vi "Update Measurement from Metadata.vi"(7 "client service_class":string, 8 "error in":errorcluster, 9 "default value":variant, 10 "metadata":T1, 11 "file refnums":refnum<vi>[](array[refnum])) -> (0 "error out":errorcluster)   [LabVIEW 2021, in "NI Measurement V2 Client Generator Runtime.lvlib"]
uses:
  NI Measurement V2 Client Generator Runtime.lvlib
  <vilib>/gRPC/Generated APIs/ni/measurementlink/measurement/v2/Measurement Service Client V2/RPC Messages/ni_measurementlink_measurement_v2_GetMetadataResponse.ctl
  <vilib>/gRPC/Generated APIs/ni/measurementlink/measurement/v2/Measurement Service Client V2/RPC Messages/ni_measurementlink_measurement_v2_MeasurementDetails.ctl
  <vilib>/gRPC/Generated APIs/ni/measurementlink/measurement/v2/Measurement Service Client V2/RPC Messages/ni_measurementlink_measurement_v2_MeasurementSignature.ctl
  <vilib>/gRPC/Generated APIs/ni/measurementlink/measurement/v2/Measurement Service Client V2/RPC Messages/ni_measurementlink_measurement_v2_ConfigurationParameter.ctl
  <vilib>/gRPC/Generated APIs/ni/measurementlink/measurement/v2/Measurement Service Client V2/RPC Messages/google_protobuf_Field_Kind.ctl
  <vilib>/gRPC/Generated APIs/ni/measurementlink/measurement/v2/Measurement Service Client V2/RPC Messages/ni_measurementlink_measurement_v2_ConfigurationParameter_AnnotationsEntry.ctl
  <vilib>/gRPC/Generated APIs/ni/measurementlink/measurement/v2/Measurement Service Client V2/RPC Messages/google_protobuf_Any.ctl
  <vilib>/gRPC/Generated APIs/ni/measurementlink/measurement/v2/Measurement Service Client V2/RPC Messages/ni_measurementlink_measurement_v2_Output.ctl
  <vilib>/gRPC/Generated APIs/ni/measurementlink/measurement/v2/Measurement Service Client V2/RPC Messages/ni_measurementlink_measurement_v2_Output_AnnotationsEntry.ctl
  <vilib>/gRPC/Generated APIs/ni/measurementlink/measurement/v2/Measurement Service Client V2/RPC Messages/ni_measurementlink_measurement_v2_UserInterfaceDetails.ctl
  <vilib>/Utility/traverseref.llb/TRef TravTarget.ctl
  Client Generator Error Strings Global.vi
  <vilib>/Utility/traverseref.llb/VI Scripting - Traverse.lvlib
  <vilib>/gRPC/Generated APIs/ni/measurementlink/measurement/v2/Measurement Service Client V2/Measurement Service Client V2.lvlib
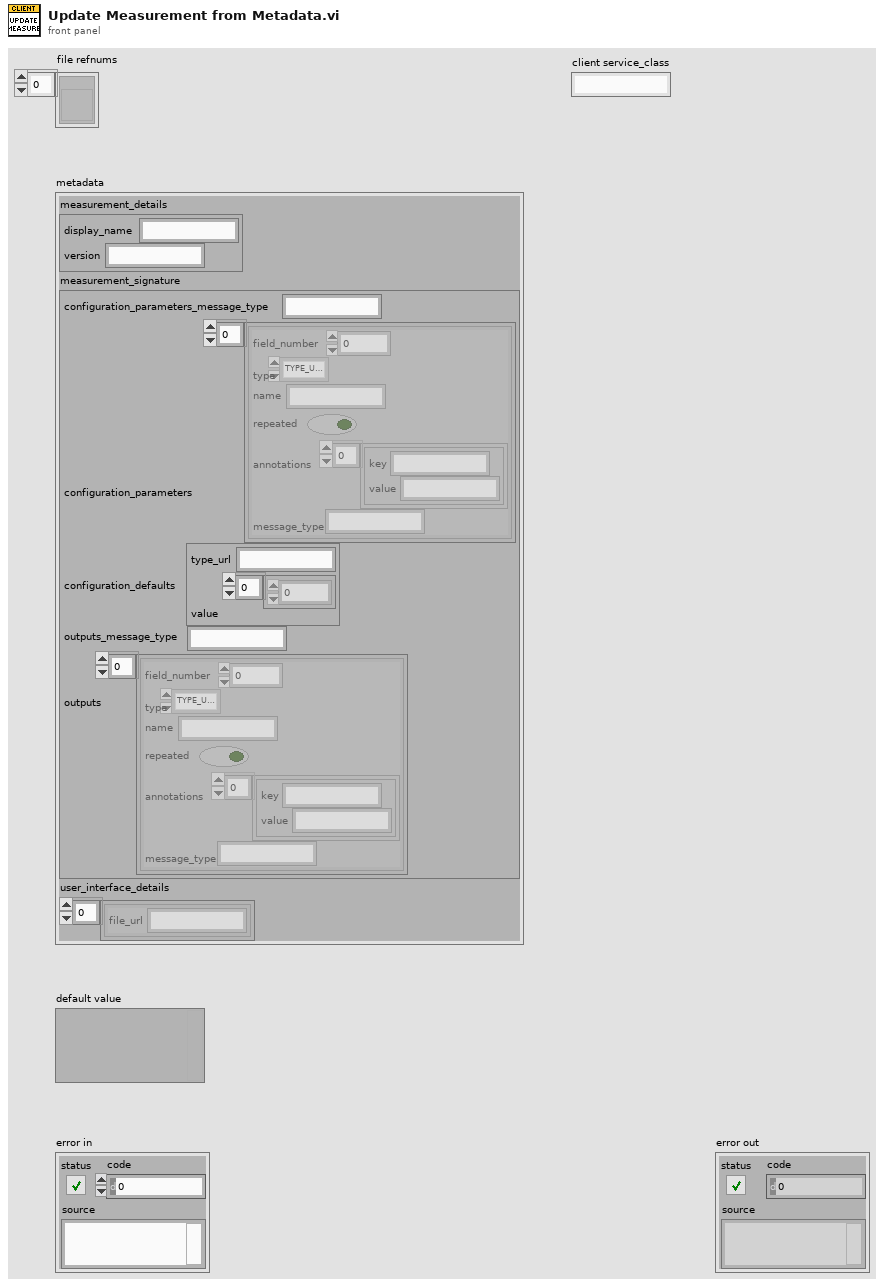
[diagram p1: front panel]
types:
  T1 = typedef "Measurement Service Client V2.lvlib/ni_measurementlink_measurement_v2_GetMetadataResponse.ctl" = cluster{"measurement_details":T2, "measurement_signature":T3, "user_interface_details":T10[]}
  T2 = typedef "Measurement Service Client V2.lvlib/ni_measurementlink_measurement_v2_MeasurementDetails.ctl" = cluster{"display_name":string, "version":string}
  T3 = typedef "Measurement Service Client V2.lvlib/ni_measurementlink_measurement_v2_MeasurementSignature.ctl" = cluster{"configuration_parameters_message_type":string, "configuration_parameters":T4[], "configuration_defaults":T7, "outputs_message_type":string, "outputs":T8[]}
  T4 = typedef "Measurement Service Client V2.lvlib/ni_measurementlink_measurement_v2_ConfigurationParameter.ctl" = cluster{"field_number":i32, "type":T5, "name":string, "repeated":bool, "annotations":T6[], "message_type":string}
  T5 = typedef "Measurement Service Client V2.lvlib/google_protobuf_Field_Kind.ctl" = enum32{"TYPE_UNKNOWN", "TYPE_DOUBLE", "TYPE_FLOAT", "TYPE_INT64", "TYPE_UINT64", "TYPE_INT32", "TYPE_FIXED64", "TYPE_FIXED32", "TYPE_BOOL", "TYPE_STRING", "TYPE_GROUP", "TYPE_MESSAGE", "TYPE_BYTES", "TYPE_UINT32", "TYPE_ENUM", "TYPE_SFIXED32", "TYPE_SFIXED64", "TYPE_SINT32", "TYPE_SINT64"}
  T6 = typedef "Measurement Service Client V2.lvlib/ni_measurementlink_measurement_v2_ConfigurationParameter_AnnotationsEntry.ctl" = cluster{"key":string, "value":string}
  T7 = typedef "Measurement Service Client V2.lvlib/google_protobuf_Any.ctl" = cluster{"type_url":string, "value":u8[]}
  T8 = typedef "Measurement Service Client V2.lvlib/ni_measurementlink_measurement_v2_Output.ctl" = cluster{"field_number":i32, "type":T5, "name":string, "repeated":bool, "annotations":T9[], "message_type":string}
  T9 = typedef "Measurement Service Client V2.lvlib/ni_measurementlink_measurement_v2_Output_AnnotationsEntry.ctl" = cluster{"key":string, "value":string}
  T10 = typedef "Measurement Service Client V2.lvlib/ni_measurementlink_measurement_v2_UserInterfaceDetails.ctl" = cluster{"file_url":string}
  T11 = typedef "TRef TravTarget.ctl" = enum16{"FP", "BD", "Other"}
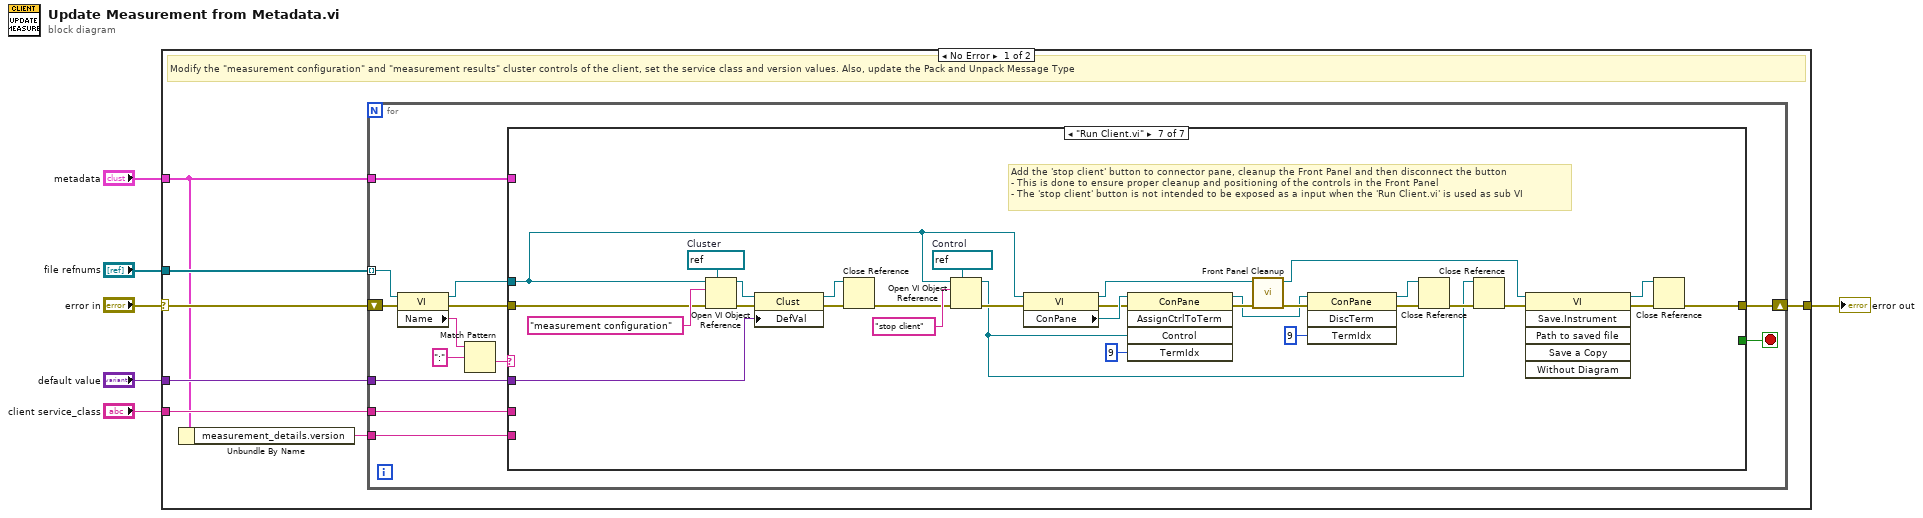
[diagram p0: block diagram]
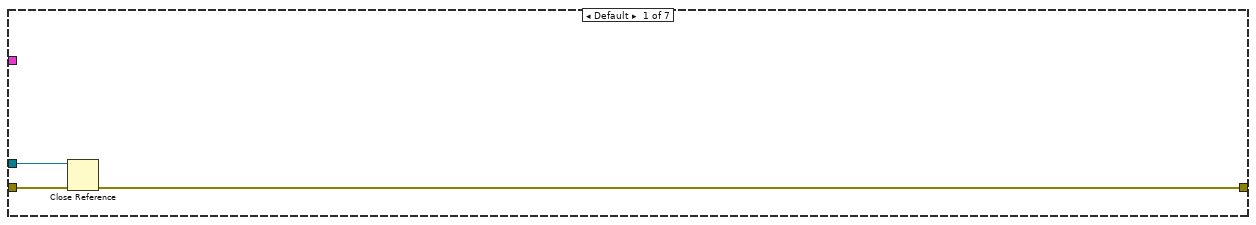
[diagram p2: hidden frame]
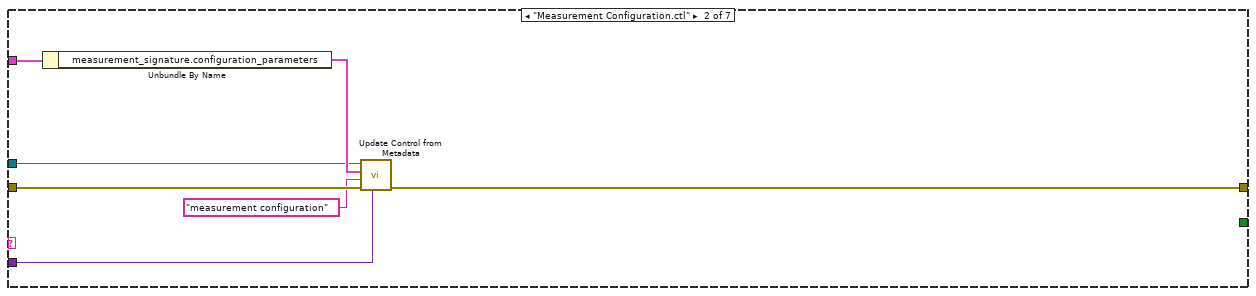
[diagram p3: hidden frame]
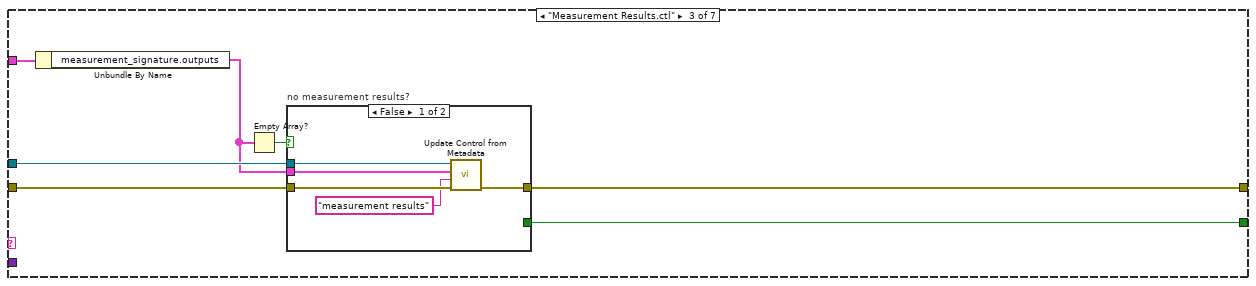
[diagram p4: hidden frame]
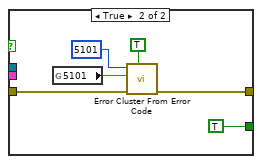
[diagram p5: hidden frame]
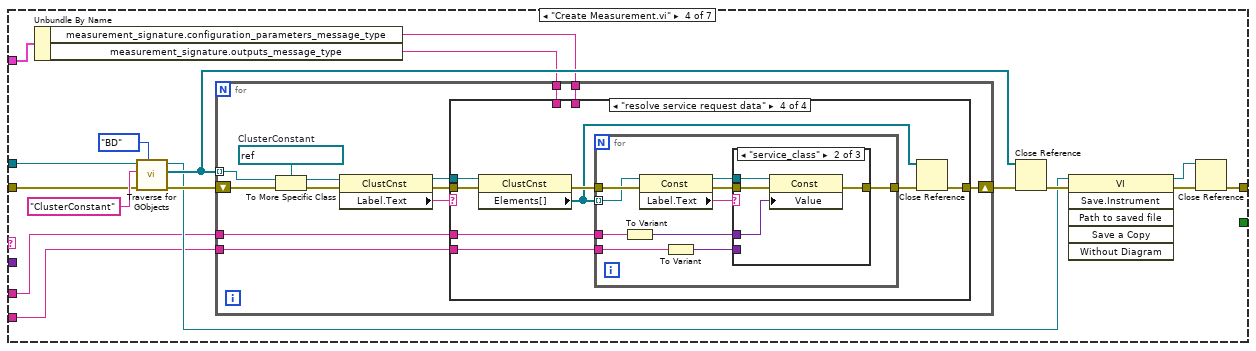
[diagram p6: hidden frame]
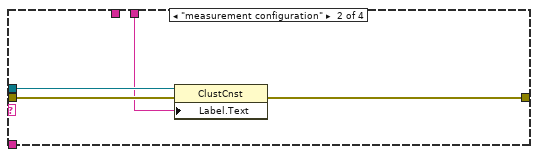
[diagram p8: hidden frame]
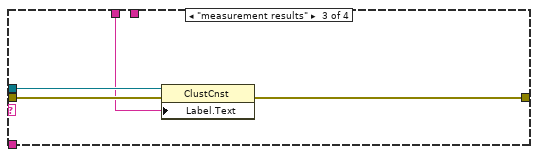
[diagram p9: hidden frame]
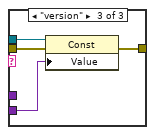
[diagram p11: hidden frame]
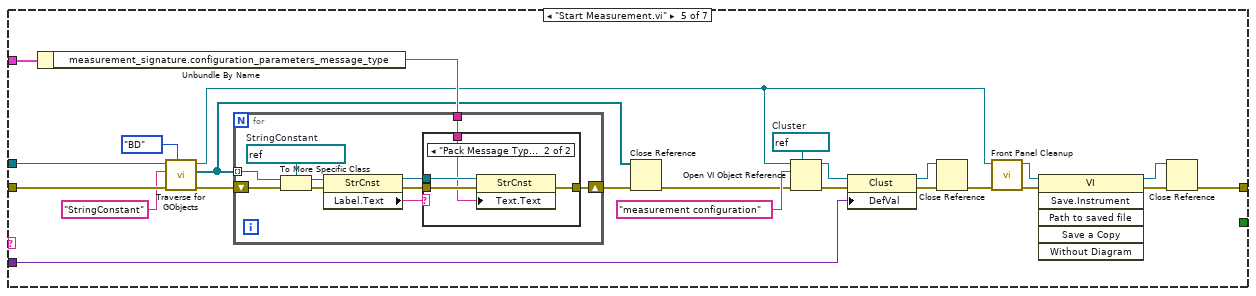
[diagram p12: hidden frame]
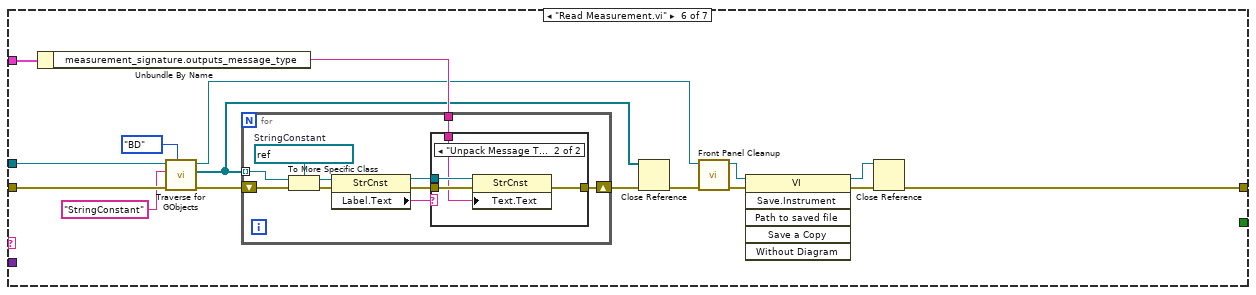
[diagram p14: hidden frame]
diagram:
  n1 = case shown="No Error" "error in" {
    selector: "error in" -> [w13 w221]
    tunnel: "client service_class" -> [w11 _]
    tunnel: "file refnums" -> [w12 _]
    tunnel: "default value" -> [w10 _]
    tunnel: "metadata" -> [w9 _]
    tunnel: [w7 w221] -> w1
    frame No Error {
      # "Modify the \"measurement configuration\" and \"measurement results\" cluster controls of the client, set the service class and version values. Also, update the Pack and Unpack Message Type"
      n2 = Unbundle By Name(w9) -> ("measurement_details.version"=w8:string)
      n3 = for {
        shift-right: [w25] -> w7
        shift-left: w13 -> [w26]
        tunnel: w12 -> [w23] mode=indexing
        tunnel: w11 -> [w20]
        tunnel: w10 -> [w19]
        tunnel: w9 -> [w18]
        tunnel: w8 -> [w17]
        stop <- w14 stop-if-true
        n4 = property class="VI"(reference=w23, error in=w26) -> (reference out=w15:refnum<vi>, error out=w24:errorcluster, "Name"=w21:string)
        n5 = Match Pattern(string=w21, regular expression=":") -> (after substring=w16:string)  [unwired: 1 in, 3 out]
        n6 = case shown="\"Run Client.vi\"" w16 {
          tunnel: w24 -> [w29 w36 w43 w60 w144 w175 w213]
          tunnel: [w28 w32 w41 w69 w121 w162 w198] -> w25
          tunnel: w15 -> [w27 w33 w42 w61 w143 w174 w206]
          tunnel: w20 -> [_ _ _ w57 _ _ _]
          tunnel: w19 -> [_ w31 _ _ w133 _ w212]
          tunnel: w18 -> [_ w30 w40 w56 w128 w167 _]
          tunnel: w17 -> [_ _ _ w55 _ _ _]
          tunnel: [_ _ w37 _ _ _ _] -> w14
          frame Default {
            n7 = Close Reference(reference=w27, error in (no error)=w29) -> (error out=w28:errorcluster)
          }
          frame "Measurement Configuration.ctl" {
            n8 = Unbundle By Name(w30) -> ("measurement_signature.configuration_parameters"=w34:T4[])
            n9 = call "Update Control from Metadata.vi"("default_value"=w31, "error in"=w36, "control name"="measurement configuration", "parameter data"=w34, "vi refnum"=w33) -> ("error out"=w32:errorcluster)  [unwired: 6 in]
          }
          frame "Measurement Results.ctl" {
            n10 = Unbundle By Name(w40) -> ("measurement_signature.outputs"=w39:T8[])
            n11 = Empty Array?(array=w39) -> (empty?=w38:bool)
            n12 = case "no measurement results?" shown="False" w38 {
              tunnel: w43 -> [w48 w51]
              tunnel: w39 -> [w46 _]
              tunnel: w42 -> [w45 _]
              tunnel: [w44 w50] -> w41
              tunnel: [_ TRUE] -> w37
              frame False {
                n13 = call "Update Control from Metadata.vi"("error in"=w48, "control name"="measurement results", "parameter data"=w46, "vi refnum"=w45) -> ("error out"=w44:errorcluster)  [unwired: 7 in]
              }
              frame True {
                n14 = global read "Client Generator Error Strings Global.vi" "5101"() -> (w53:string)
                n15 = call <vilib>:"Error Cluster From Error Code.vi"("show call chain? (False)"=TRUE, "error in (no error)"=w51, "error message (\"\")"=w53, "error code (0)"=5101) -> ("error out"=w50:errorcluster)  [unwired: 5 in]
              }
            }
          }
          frame "Create Measurement.vi" {
            n16 = Unbundle By Name(w56) -> ("measurement_signature.configuration_parameters_message_type"=w64:string, "measurement_signature.outputs_message_type"=w63:string)
            n17 = call <vilib>:"Traverse for GObjects.vi"("Traverse Target"=TRef_TravTarget."BD", "error in (no error)"=w60, "Class Name"="ClusterConstant", "VI Refnum"=w61) -> ("error out"=w68:errorcluster, "References"=w66:refnum<vi>[], "dup VI Refnum"=w58:refnum<vi>)  [unwired: 4 in, 1 out]
            n18 = for {
              shift-right: [w79] -> w62
              shift-left: w68 -> [w84]
              tunnel: w66 -> [w82] mode=indexing
              tunnel: w64 -> [w77]
              tunnel: w63 -> [w76]
              tunnel: w57 -> [w73]
              tunnel: w55 -> [w72]
              w75 = refnum<vi> refnum  # ClusterConstant
              n19 = To More Specific Class(target class=w75, reference=w82, error in=w84) -> (specific class reference=w81:refnum<vi>, error out=w83:errorcluster)
              n20 = property class="ClustCnst"(reference=w81, error in=w83) -> (reference out=w78:refnum<vi>, error out=w80:errorcluster, "Label.Text"=w74:string)
              n21 = case shown="\"resolve service request data\"" w74 {
                tunnel: [w85 w88 w92 w97] -> w79
                tunnel: w80 -> [w85 w89 w93 w101]
                tunnel: w78 -> [_ w87 w91 w100]
                tunnel: w77 -> [_ w86 _ _]
                tunnel: w76 -> [_ _ w90 _]
                tunnel: w73 -> [_ _ _ w95]
                tunnel: w72 -> [_ _ _ w94]
                frame Default {
                }
                frame "measurement configuration" {
                  n22 = property class="ClustCnst"(reference=w87, error in=w89, "Label.Text"=w86) -> (error out=w88:errorcluster)  [unwired: 1 out]
                }
                frame "measurement results" {
                  n23 = property class="ClustCnst"(reference=w91, error in=w93, "Label.Text"=w90) -> (error out=w92:errorcluster)  [unwired: 1 out]
                }
                frame "resolve service request data" {
                  n24 = property class="ClustCnst"(reference=w100, error in=w101) -> (error out=w99:errorcluster, "Elements[]"=w96:refnum<vi>[])  [unwired: 1 out]
                  n25 = for {
                    tunnel: w96 -> [w110] mode=indexing
                    tunnel: w99 -> [w111]
                    tunnel: [w106] -> w98
                    tunnel: w95 -> [w103]
                    tunnel: w94 -> [w102]
                    n26 = To Variant(anything=w103) -> (Variant=w104:variant)
                    n27 = property class="Const"(reference=w110, error in=w111) -> (reference out=w107:refnum<vi>, error out=w108:errorcluster, "Label.Text"=w109:string)
                    n28 = To Variant(anything=w102) -> (Variant=w105:variant)
                    n29 = case shown="\"service_class\"" w109 {
                      tunnel: w108 -> [w112 w116 w120]
                      tunnel: w107 -> [_ w115 w119]
                      tunnel: [w112 w114 w118] -> w106
                      tunnel: w105 -> [_ _ w117]
                      tunnel: w104 -> [_ w113 _]
                      frame Default {
                      }
                      frame "service_class" {
                        n30 = property class="Const"(reference=w115, error in=w116, "Value"=w113) -> (error out=w114:errorcluster)  [unwired: 1 out]
                      }
                      frame "version" {
                        n31 = property class="Const"(reference=w119, error in=w120, "Value"=w117) -> (error out=w118:errorcluster)  [unwired: 1 out]
                      }
                    }
                  }
                  n32 = Close Reference(reference=w96, error in (no error)=w98) -> (error out=w97:errorcluster)
                }
              }
            }
            n33 = Close Reference(reference=w66, error in (no error)=w62) -> (error out=w59:errorcluster)
            n34 = invoke class="VI" method="Save.Instrument"(reference=w58, error in=w59) -> (reference out=w71:refnum<vi>, error out=w70:errorcluster)  [unwired: 4 in, 4 out]
            n35 = Close Reference(reference=w71, error in (no error)=w70) -> (error out=w69:errorcluster)
          }
          frame "Start Measurement.vi" {
            w136 = refnum<vi> refnum  # Cluster
            n36 = Unbundle By Name(w128) -> ("measurement_signature.configuration_parameters_message_type"=w139:string)
            n37 = call <vilib>:"Traverse for GObjects.vi"("Traverse Target"=TRef_TravTarget."BD", "error in (no error)"=w144, "Class Name"="StringConstant", "VI Refnum"=w143) -> ("error out"=w140:errorcluster, "References"=w129:refnum<vi>[], "dup VI Refnum"=w123:refnum<vi>)  [unwired: 4 in, 1 out]
            n38 = for {
              shift-right: [w154] -> w138
              shift-left: w140 -> [w153]
              tunnel: w129 -> [w151] mode=indexing
              tunnel: w139 -> [w145]
              w150 = refnum<vi> refnum  # StringConstant
              n39 = To More Specific Class(target class=w150, reference=w151, error in=w153) -> (specific class reference=w148:refnum<vi>, error out=w152:errorcluster)
              n40 = property class="StrCnst"(reference=w148, error in=w152) -> (reference out=w147:refnum<vi>, error out=w149:errorcluster, "Label.Text"=w146:string)
              n41 = case shown="\"Pack Message Type\"" w146 {
                tunnel: [w155 w159] -> w154
                tunnel: w149 -> [w155 w158]
                tunnel: w147 -> [_ w157]
                tunnel: w145 -> [_ w156]
                frame Default {
                }
                frame "Pack Message Type" {
                  n42 = property class="StrCnst"(reference=w157, error in=w158, "Text.Text"=w156) -> (error out=w159:errorcluster)  [unwired: 1 out]
                }
              }
            }
            n43 = Close Reference(reference=w129, error in (no error)=w138) -> (error out=w130:errorcluster)
            n44 = Open VI Object Reference(7:w136, 8:w130, 10:"measurement configuration" ("name/order"), 11:w123) -> (0:w137:errorcluster, 3:w134:refnum<vi>)
            n45 = property class="Clust"(reference=w134, error in=w137, "DefVal"=w133) -> (reference out=w132:refnum<vi>, error out=w135:errorcluster)
            n46 = Close Reference(reference=w132, error in (no error)=w135) -> (error out=w122:errorcluster)
            n47 = call "Front Panel Cleanup.vi"("error in"=w122, "vi refnum"=w123) -> ("error out"=w126:errorcluster, "vi refnum out"=w127:refnum<vi>)  [unwired: 8 in]
            n48 = invoke class="VI" method="Save.Instrument"(reference=w127, error in=w126) -> (reference out=w124:refnum<vi>, error out=w125:errorcluster)  [unwired: 4 in, 4 out]
            n49 = Close Reference(reference=w124, error in (no error)=w125) -> (error out=w121:errorcluster)
          }
          frame "Read Measurement.vi" {
            n50 = Unbundle By Name(w167) -> ("measurement_signature.outputs_message_type"=w170:string)
            n51 = call <vilib>:"Traverse for GObjects.vi"("Traverse Target"=TRef_TravTarget."BD", "error in (no error)"=w175, "Class Name"="StringConstant", "VI Refnum"=w174) -> ("error out"=w171:errorcluster, "References"=w168:refnum<vi>[], "dup VI Refnum"=w160:refnum<vi>)  [unwired: 4 in, 1 out]
            n52 = for {
              shift-right: [w185] -> w169
              shift-left: w171 -> [w184]
              tunnel: w168 -> [w182] mode=indexing
              tunnel: w170 -> [w176]
              w181 = refnum<vi> refnum  # StringConstant
              n53 = To More Specific Class(target class=w181, reference=w182, error in=w184) -> (specific class reference=w179:refnum<vi>, error out=w183:errorcluster)
              n54 = property class="StrCnst"(reference=w179, error in=w183) -> (reference out=w178:refnum<vi>, error out=w180:errorcluster, "Label.Text"=w177:string)
              n55 = case shown="\"Unpack Message Type\"" w177 {
                tunnel: [w186 w190] -> w185
                tunnel: w180 -> [w186 w189]
                tunnel: w178 -> [_ w188]
                tunnel: w176 -> [_ w187]
                frame Default {
                }
                frame "Unpack Message Type" {
                  n56 = property class="StrCnst"(reference=w188, error in=w189, "Text.Text"=w187) -> (error out=w190:errorcluster)  [unwired: 1 out]
                }
              }
            }
            n57 = Close Reference(reference=w168, error in (no error)=w169) -> (error out=w161:errorcluster)
            n58 = call "Front Panel Cleanup.vi"("error in"=w161, "vi refnum"=w160) -> ("error out"=w165:errorcluster, "vi refnum out"=w166:refnum<vi>)  [unwired: 8 in]
            n59 = invoke class="VI" method="Save.Instrument"(reference=w166, error in=w165) -> (reference out=w163:refnum<vi>, error out=w164:errorcluster)  [unwired: 4 in, 4 out]
            n60 = Close Reference(reference=w163, error in (no error)=w164) -> (error out=w162:errorcluster)
          }
          frame "Run Client.vi" {
            w194 = refnum<vi> refnum  # Control
            w218 = refnum<vi> refnum  # Cluster
            # "Add the 'stop client' button to connector pane, cleanup the Front Panel and then disconnect the button\n- This is done to ensure proper cleanup and positioning of the controls in the Front Panel\n- The 'stop client' button is not intended to be exposed as a input when the 'Run Client.vi' is used as sub VI"
            n61 = Open VI Object Reference(7:w218, 8:w213, 10:"measurement configuration" ("name/order"), 11:w206) -> (0:w219:errorcluster, 3:w216:refnum<vi>)
            n62 = property class="Clust"(reference=w216, error in=w219, "DefVal"=w212) -> (reference out=w215:refnum<vi>, error out=w217:errorcluster)
            n63 = Close Reference(reference=w215, error in (no error)=w217) -> (error out=w207:errorcluster)
            n64 = Open VI Object Reference(7:w194, 8:w207, 10:"stop client" ("name/order"), 11:w206) -> (0:w208:errorcluster, 3:w192:refnum<vi>)
            n65 = property class="VI"(reference=w206, error in=w208) -> (reference out=w205:refnum<vi>, error out=w209:errorcluster, "ConPane"=w210:refnum<vi>)
            n66 = invoke class="ConPane" method="AssignCtrlToTerm"(reference=w210, error in=w209, "Control"=w192, "TermIdx"=u32 9 ("Terminal Index")) -> (reference out=w202:refnum<vi>, error out=w204:errorcluster)  [unwired: 1 in, 3 out]
            n67 = call "Front Panel Cleanup.vi"("error in"=w204, "vi refnum"=w205) -> ("error out"=w203:errorcluster, "vi refnum out"=w199:refnum<vi>)  [unwired: 8 in]
            n68 = invoke class="ConPane" method="DiscTerm"(reference=w202, error in=w203, "TermIdx"=u32 9 ("Terminal Index")) -> (reference out=w191:refnum<vi>, error out=w201:errorcluster)  [unwired: 1 in, 2 out]
            n69 = Close Reference(reference=w191, error in (no error)=w201) -> (error out=w200:errorcluster)
            n70 = Close Reference(reference=w192, error in (no error)=w200) -> (error out=w193:errorcluster)
            n71 = invoke class="VI" method="Save.Instrument"(reference=w199, error in=w193) -> (reference out=w220:refnum<vi>, error out=w197:errorcluster)  [unwired: 4 in, 4 out]
            n72 = Close Reference(reference=w220, error in (no error)=w197) -> (error out=w198:errorcluster)
          }
        }
      }
    }
    frame Error {
      # "Pass"
    }
  }
  "error out" <- w1
